vi "Swerve Balance To Level PID.vi"(7 "Yaw Data":T1, 8 "Position ft":dbl, 11 "Tilt PID Config":T3={"Gains"={"P"=1.0, "I"=0.01, "D"=0.0, "F"=0.0}, "Error Allowed"={"High"=0.1, "Low"=-0.1}, "I Zone"={"High"=10.0, "Low"=-10.0}, "Max Out"={"FWD"=100.0, "REV"=-100.0}, "Max I Accu"={"High"=0.0, "Low"=0.0}, "CL Ramp Rate (S)"=0.0} {"Max I Accu"."Low" format="%#.8f"; "Max I Accu"."High" format="%#.8f"; "Gains"."F" format="%#.8f"; "Gains"."D" format="%#.8f"; "Gains"."I" format="%#.8f"; "Gains"."P" format="%#.8f"; "Error Allowed"."Low" format="%#.8f"; "Error Allowed"."High" format="%#.8f"; "I Zone"."Low" format="%#.8f"; "I Zone"."High" format="%#.8f"; "Max Out"."REV" format="%.2f"; "Max Out"."FWD" format="%.2f"}) -> (1 "Balanced":bool, 3 "Output Cluster Out":T7 {"Angle" scale format="%.3f"; "Velocity" scale=-1.0..1.0 scale format="%.1f"}, 5 "Lock":bool)   [LabVIEW 2023, in "Thor-SwerveDrive_ACT.lvlib"]
uses:
  Thor-SwerveDrive_ACT.lvlib
  Shared Code/TypeDefs/Dial_Compase heading unit circle CCW positive.ctl
  Shared Code/TypeDefs/Level_Velocity plus-minus 1.ctl
  Shared Code/TypeDefs/Cluster_Module Velocity-Direction-Rotations.ctl
  Shared Code/TypeDefs/Cluster_PID Gains.ctl
  Shared Code/TypeDefs/Cluster_High-Low.ctl
  Shared Code/TypeDefs/Cluster_PID Config.ctl
  Shared Code/TypeDefs/Cluster_FWD  REV Values.ctl
  Type Defs/Cluster_Pigeon Tilt Data.ctl
  Shared Code/TypeDefs/ENUM_Tilt State.ctl
panel:
  in  "% out max":dbl
  out "Time Remaining":dbl
  out "not moving":bool
  out "inrange":bool
  out "Error Out":dbl
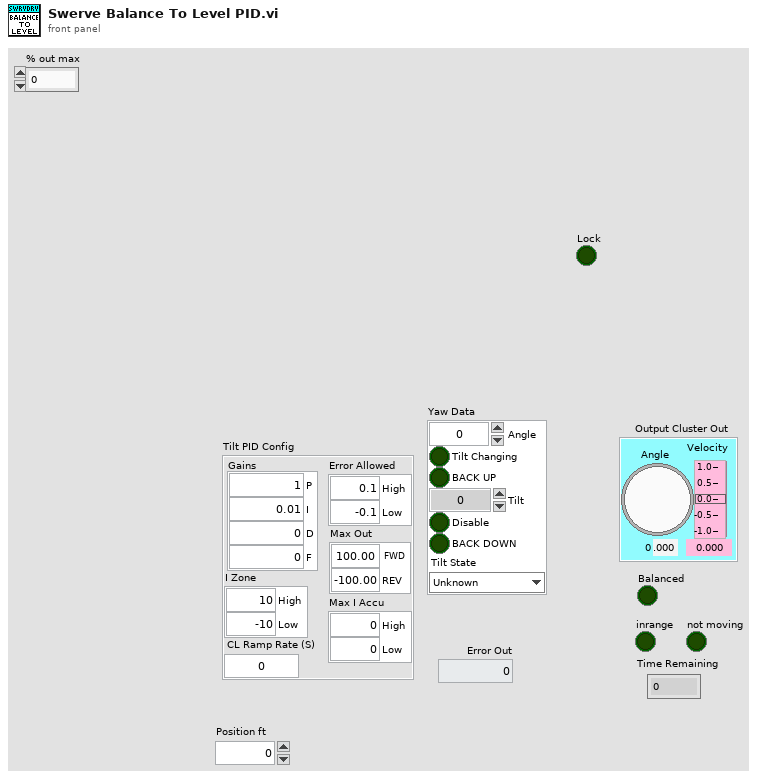
[diagram p1: front panel]
types:
  T1 = typedef "Cluster_Pigeon Tilt Data.ctl" = cluster{"Angle":dbl, "Tilt Changing":bool, "BACK UP":bool, "Tilt":dbl, "Disable":bool, "BACK DOWN":bool, "Tilt State":T2}
  T2 = typedef "ENUM_Tilt State.ctl" = enum16{"Unknown", "Level", "Angle UP from Level", "Level from Angle Up", "Angle Down from Level", "Level from Angle Down"}
  T3 = typedef "Cluster_PID Config.ctl" = cluster{"Gains":T4, "Error Allowed":T5, "I Zone":T5, "Max Out":T6, "Max I Accu":T5, "CL Ramp Rate (S)":dbl}
  T4 = typedef "Cluster_PID Gains.ctl" = cluster{"P":dbl, "I":dbl, "D":dbl, "F":dbl}
  T5 = typedef "Cluster_High-Low.ctl" = cluster{"High":dbl, "Low":dbl}
  T6 = typedef "Cluster_FWD  REV Values.ctl" = cluster{"FWD":dbl, "REV":dbl}
  T7 = typedef "Cluster_Module Velocity-Direction-Rotations.ctl" = cluster{"Velocity":T8, "Angle":T9, "Rotations Count":dbl}
  T8 = typedef "Level_Velocity plus-minus 1.ctl" = dbl
  T9 = typedef "Dial_Compase heading unit circle CCW positive.ctl" = dbl
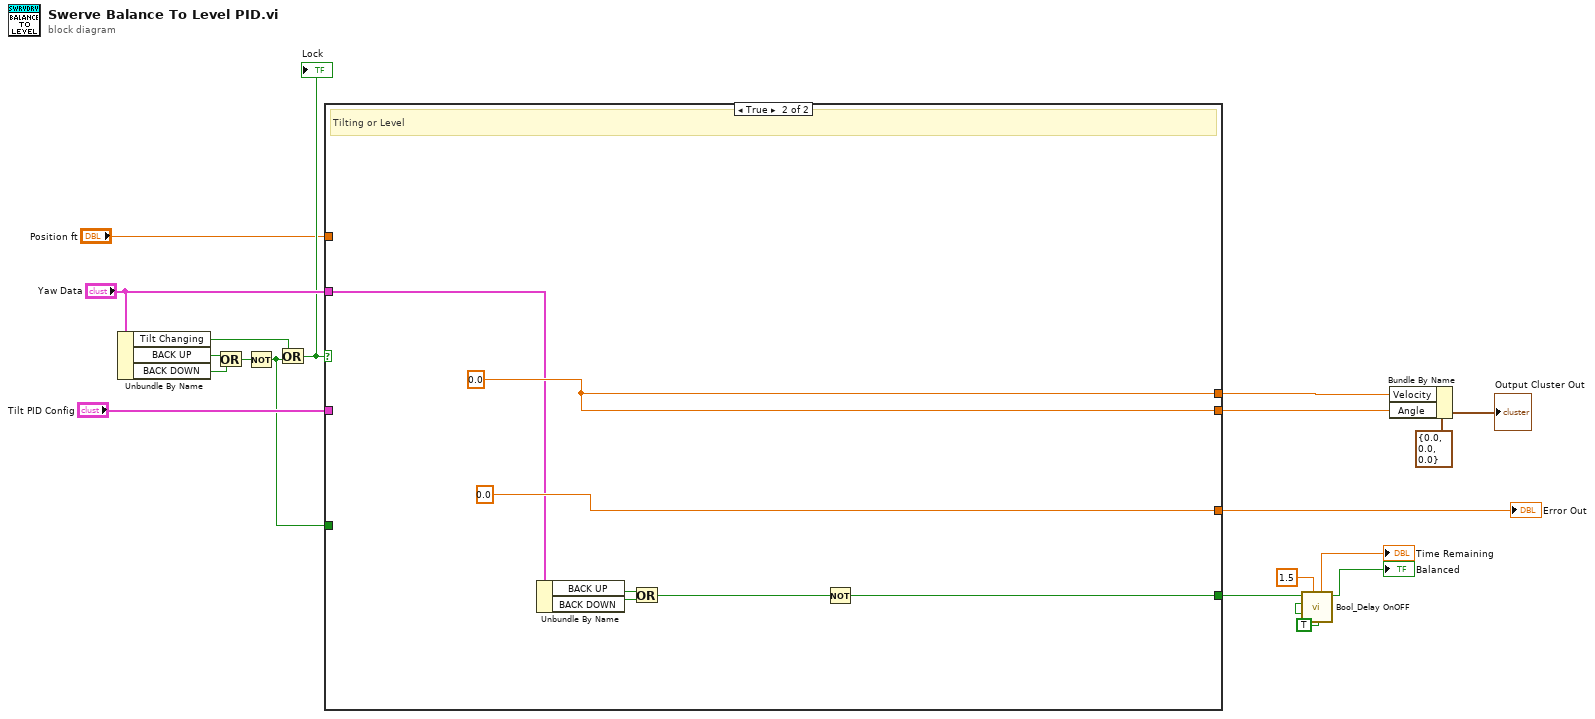
[diagram p0: block diagram]
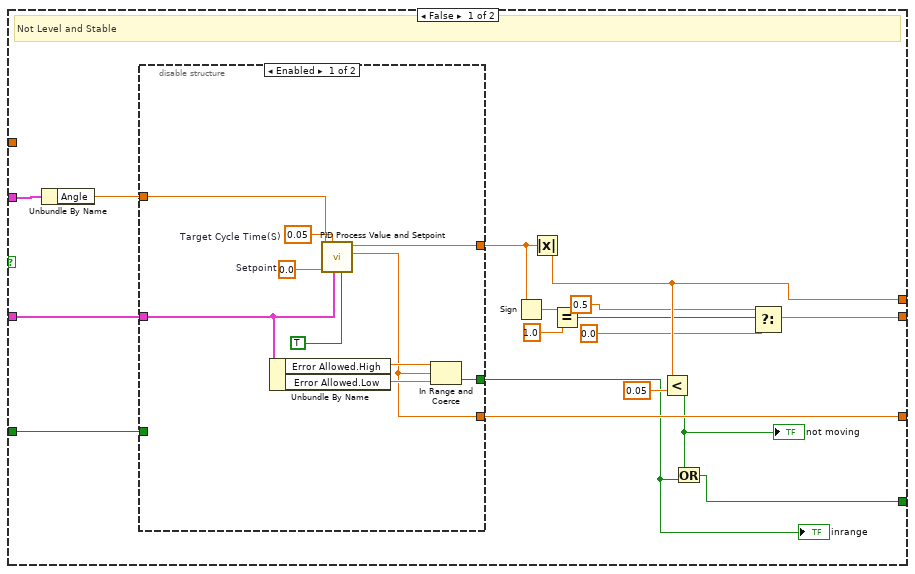
[diagram p2: hidden frame]
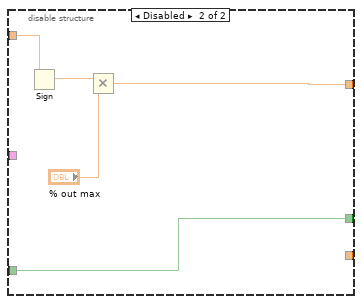
[diagram p3: hidden frame]
diagram:
  n1 = Unbundle By Name("Yaw Data") -> ("Tilt Changing"=w5:bool, "BACK UP"=w8:bool, "BACK DOWN"=w6:bool)
  n2 = Or(x=w8, y=w6) -> (x .or. y?=w7:bool)
  n3 = Not(x=w7) -> (.not. x?=w2:bool)
  n4 = Or(x=w5, y=w2) -> (x .or. y?=w3:bool)
  "Lock" <- w3
  n5 = case shown="True" w3 {
    tunnel: [w36 w58] -> w18
    tunnel: [w35 w58] -> w16
    tunnel: "Tilt PID Config" -> [w34 _]
    tunnel: [w27 0.0 ("Error Out")] -> w14
    tunnel: [w23 w56] -> w11
    tunnel: "Yaw Data" -> [w22 w55]
    tunnel: w2 -> [w20 _]
    tunnel: "Position ft" -> [_ _]
    frame False {
      # "Not Level and Stable"
      n6 = Unbundle By Name(w22) -> ("Angle"=w21:dbl)
      n7 = disable-structure shown="Enabled" {
        disable-tunnel: w34 -> [w46 _]
        disable-tunnel: [w45 w48] -> w28
        disable-tunnel: [w39 _] -> w27
        disable-tunnel: [w38 w47] -> w25
        disable-tunnel: w21 -> [w37 w51]
        disable-tunnel: w20 -> [_ w47]
        frame Enabled {
          w43 = 0.05  # Target Cycle Time(S)
          w44 = 0.0  # Setpoint
          n8 = Unbundle By Name(w46) -> ("Error Allowed.High"=w41:dbl, "Error Allowed.Low"=w40:dbl)
          n9 = call "PID Process Value and Setpoint.vi"("Allowable Error Disables Accumulator"=TRUE, "PID Config"=w46, "Target Cycle Time(S)"=w43, "Setpoint"=w44, "Process Variable"=w37) -> ("Error Out"=w39:dbl, "Output Out"=w45:dbl)  [unwired: 3 in, 2 out]
          n10 = In Range and Coerce(upper limit=w41, x=w39, lower limit=w40) -> (In Range?=w38:bool)  [unwired: 1 out]
        }
        frame Disabled {
          n11 = Sign(1:w51) -> (0:w50:dbl)
          n12 = Multiply(x=w50, y="% out max") -> (x*y=w48:dbl)
        }
      }
      "inrange" <- w25
      n13 = Sign(1:w28) -> (0:w33:dbl)
      n14 = Absolute Value(x=w28) -> (abs(x)=w35:dbl)
      n15 = Equal?(x=w33, y=1.0) -> (x = y?=w31:bool)
      n16 = Less?(x=w35, y=0.05) -> (x < y?=w24:bool)
      "not moving" <- w24
      n17 = Or(x=w24, y=w25) -> (x .or. y?=w23:bool)
      n18 = Select(t=0.5, s=w31, f=0.0) -> (s? t:f=w36:dbl)
    }
    frame True {
      w58 = 0.0
      # "Tilting or Level"
      n19 = Unbundle By Name(w55) -> ("BACK UP"=w54:bool, "BACK DOWN"=w53:bool)
      n20 = Or(x=w54, y=w53) -> (x .or. y?=w52:bool)
      n21 = Not(x=w52) -> (.not. x?=w56:bool)
    }
  }
  "Error Out" <- w14
  n22 = call "Bool_Delay OnOFF.vi"("Delay Time(S)"=1.5, "Delay On(t) Off(f)"=TRUE, "Input"=w11) -> ("Output"=→"Balanced":bool, "Time Remaining"=→"Time Remaining":dbl)  [unwired: 7 in]
  n23 = Bundle By Name(cluster=T7 {"Velocity"=0.0, "Angle"=0.0, "Rotations Count"=0.0} ("Polar Out"), "Velocity"=w16, "Angle"=w18) -> (→"Output Cluster Out":T7)
